vi "Estrai soglie.vi"(8 "error in (no error)":errorcluster, 10 "element":refnum<vi>) -> (0 "error out":errorcluster, 2 "Array soglie":T1(array[cluster]))   [LabVIEW 2019]
uses:
  <vilib>/Utility/file.llb/Read Delimited Spreadsheet (string).vi
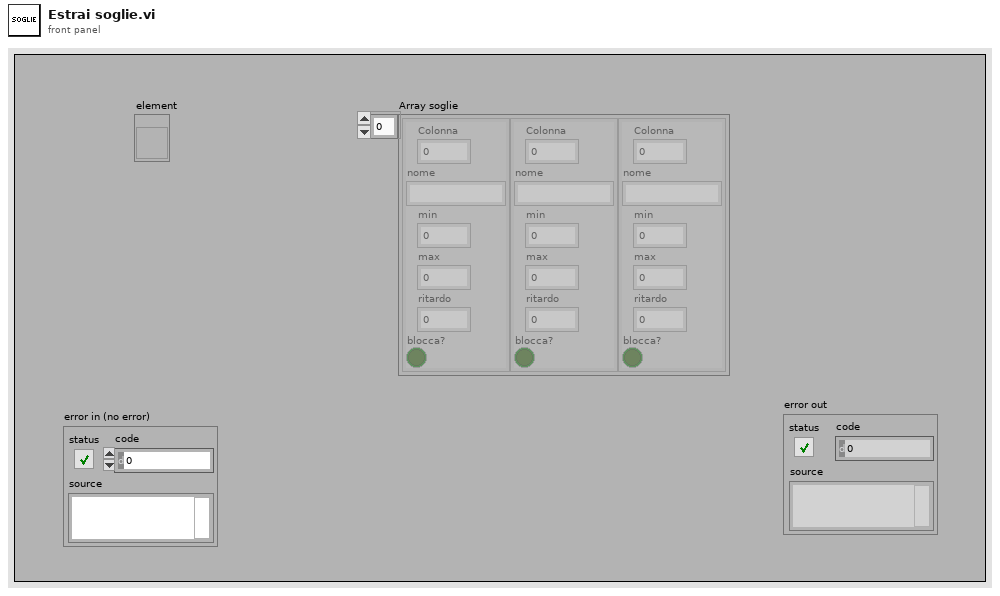
[diagram p1: front panel]
types:
  T1 = cluster{"Colonna":i16, "nome":string, "min":dbl, "max":dbl, "ritardo":dbl, "blocca?":bool}[]
  T2 = cluster{"Colonna":i16, "nome":string, "min":dbl, "max":dbl, "ritardo":dbl, "blocca?":bool}
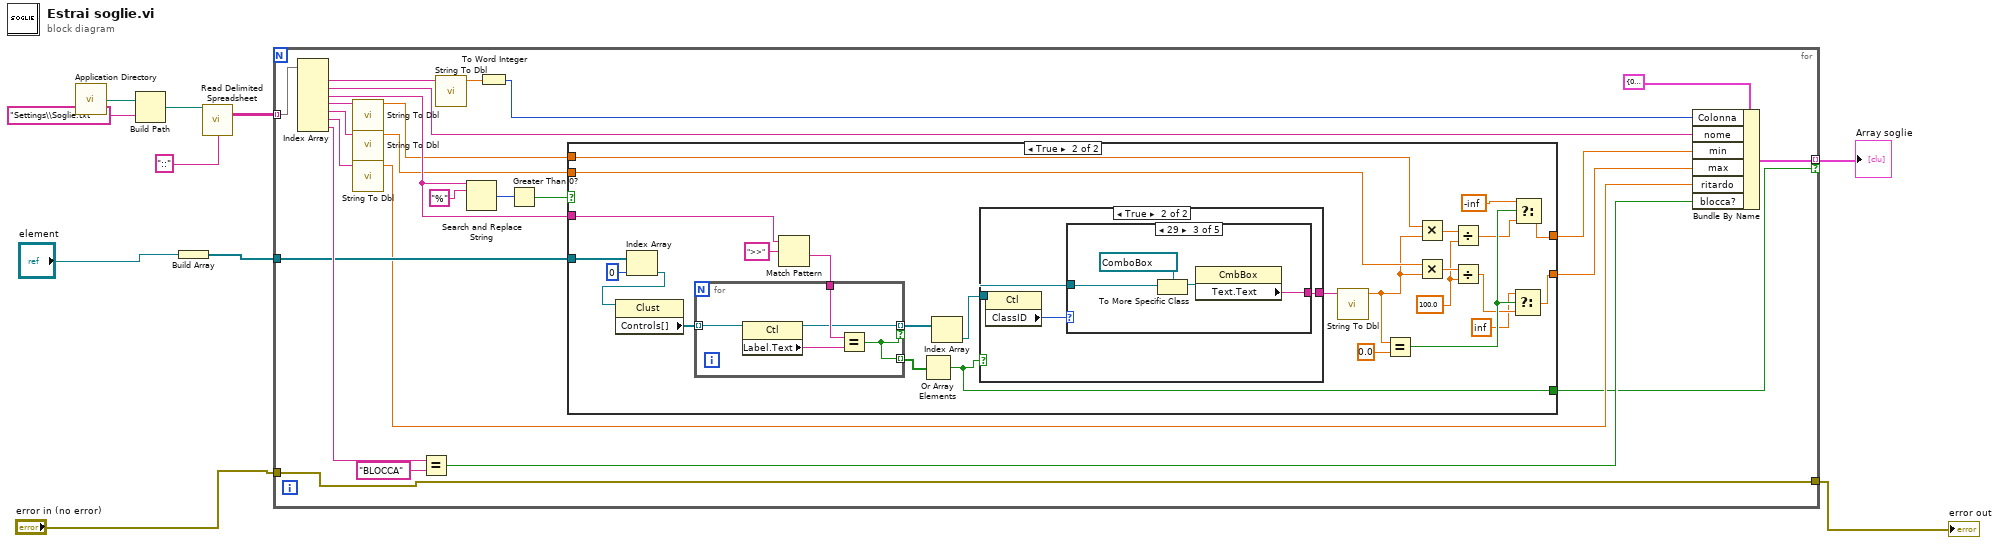
[diagram p0: block diagram]
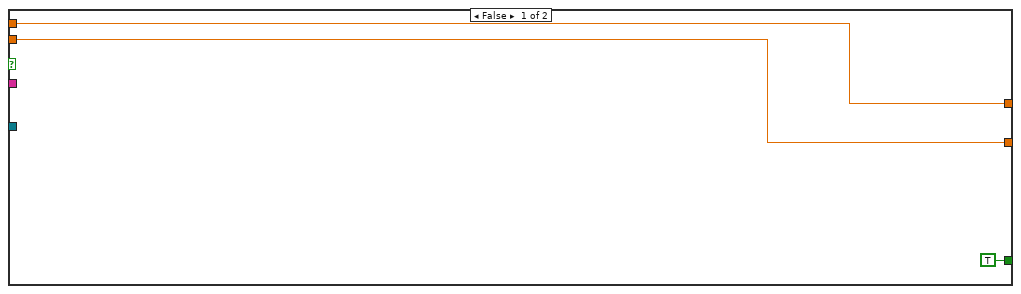
[diagram p2: hidden frame]
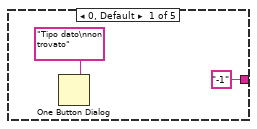
[diagram p4: hidden frame]
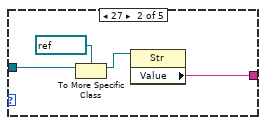
[diagram p5: hidden frame]
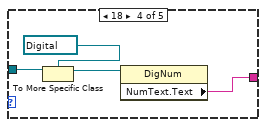
[diagram p6: hidden frame]
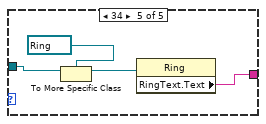
[diagram p7: hidden frame]
diagram:
  n1 = call <vilib>:"Application Directory.vi"() -> ("Application Directory"=w6:path)
  n2 = Build Path(base path=w6, name or relative path="Settings\\Soglie.txt") -> (appended path=w5:path)
  n3 = Build Array("element") -> (w10:refnum<vi>[])
  n4 = call-poly <vilib>:"Read Delimited Spreadsheet.vi"("file path (dialog if empty)"=w5, "delimiter (\\t)"="::" ("delimiter (\\t)")) -> ("all rows"=w9:string[][])  [unwired: 8 in, 5 out]
  n5 = for {
    tunnel: w9 -> [w35] mode=indexing
    tunnel: w10 -> [w24]
    tunnel: [w13] -> w4 mode=indexing if=w12
    tunnel: "error in (no error)" -> [w11]
    tunnel: [w11] -> w1
    n6 = Index Array(array=w35) -> (element #1=w34:string, element #2=w18:string, element #3=w23:string, element #4=w30:string, element #5=w29:string, element #6=w28:string, element #7=w27:string)  [unwired: 7 in]
    n7 = call "String To Dbl.vi"("String"=w30) -> ("Numeric"=w22:dbl)  [unwired: 10 in]
    n8 = call "String To Dbl.vi"("String"=w29) -> ("Numeric"=w21:dbl)  [unwired: 10 in]
    n9 = call "String To Dbl.vi"("String"=w28) -> ("Numeric"=w15:dbl)  [unwired: 10 in]
    n10 = Equal?(x=w27, y="BLOCCA") -> (x = y?=w14:bool)
    n11 = call "String To Dbl.vi"("String"=w34) -> ("Numeric"=w33:dbl)  [unwired: 10 in]
    n12 = Search and Replace String(input string=w23, search string="%") -> (number of replacements=w31:i32)  [unwired: 6 in, 3 out]
    n13 = To Word Integer(number=w33) -> (16bit integer=w19:i16)
    n14 = Greater Than 0?(x=w31) -> (x > 0?=w25:bool)
    n15 = case shown="True" w25 {
      tunnel: w24 -> [_ w64]
      tunnel: w23 -> [_ w42]
      tunnel: [w38 w45] -> w17
      tunnel: [w37 w46] -> w16
      tunnel: w22 -> [w38 w55]
      tunnel: w21 -> [w37 w54]
      tunnel: [TRUE w39] -> w12
      frame False {
      }
      frame True {
        w56 = 100.0 ("y")
        n16 = Index Array(array=w64, index=0) -> (element=w63:refnum<vi>)
        n17 = property class="Clust"(reference=w63) -> ("Controls[]"=w62:refnum<vi>[])  [unwired: 1 in, 2 out]
        n18 = Match Pattern(string=w42, regular expression=">>") -> (after substring=w41:string)  [unwired: 1 in, 3 out]
        n19 = for {
          tunnel: w62 -> [w90] mode=indexing
          tunnel: w41 -> [w88]
          tunnel: [w87] -> w61 mode=indexing if=w86
          tunnel: [w86] -> w40 mode=indexing
          n20 = property class="Ctl"(reference=w90) -> (reference out=w87:refnum<vi>, "Label.Text"=w89:string)  [unwired: 1 in, 1 out]
          n21 = Equal?(x=w88, y=w89) -> (x = y?=w86:bool)
        }
        n22 = Or Array Elements(Boolean array=w40) -> (logical OR=w39:bool)
        n23 = Index Array(array=w61) -> (element=w60:refnum<vi>)  [unwired: 1 in]
        n24 = case shown="True" w39 {
          tunnel: w60 -> [_ w67]
          tunnel: [_ w65] -> w59
          frame False {
          }
          frame True {
            n25 = property class="Ctl"(reference=w67) -> ("ClassID"=w66:u32)  [unwired: 1 in, 2 out]
            n26 = case shown="29" w66 {
              tunnel: w67 -> [_ w72 w75 w81 w84]
              tunnel: ["-1" ("RingText.Text") w70 w74 w78 w82] -> w65
              frame 0, Default {
                n27 = One Button Dialog(message="Tipo dato\nnon trovato") -> ()  [unwired: 1 in, 1 out]
              }
              frame 27 {
                n28 = To More Specific Class(target class=refnum<vi> refnum ("String"), reference=w72) -> (specific class reference=w71:refnum<vi>)  [unwired: 1 in, 1 out]
                n29 = property class="Str"(reference=w71) -> ("Value"=w70:string)  [unwired: 1 in, 2 out]
              }
              frame 29 {
                n30 = To More Specific Class(target class=refnum<vi> refnum ("String"), reference=w75) -> (specific class reference=w76:refnum<vi>)  [unwired: 1 in, 1 out]
                n31 = property class="CmbBox"(reference=w76) -> ("Text.Text"=w74:string)  [unwired: 1 in, 2 out]
              }
              frame 18 {
                n32 = To More Specific Class(target class=refnum<vi> refnum ("Numeric Control"), reference=w81) -> (specific class reference=w79:refnum<vi>)  [unwired: 1 in, 1 out]
                n33 = property class="DigNum"(reference=w79) -> ("NumText.Text"=w78:string)  [unwired: 1 in, 2 out]
              }
              frame 34 {
                n34 = To More Specific Class(target class=refnum<vi> refnum ("Menu Ring"), reference=w84) -> (specific class reference=w83:refnum<vi>)  [unwired: 1 in, 1 out]
                n35 = property class="Ring"(reference=w83) -> ("RingText.Text"=w82:string)  [unwired: 1 in, 2 out]
              }
            }
          }
        }
        n36 = call "String To Dbl.vi"("String"=w59) -> ("Numeric"=w53:dbl)  [unwired: 10 in]
        n37 = Equal?(x=w53, y=0.0) -> (x = y?=w51:bool)
        n38 = Multiply(x=w55, y=w53) -> (x*y=w58:dbl)
        n39 = Multiply(x=w54, y=w53) -> (x*y=w57:dbl)
        n40 = Divide(x=w58, y=w56) -> (x/y=w49:dbl)
        n41 = Divide(x=w57, y=w56) -> (x/y=w50:dbl)
        n42 = Select(t=inf ("y"), s=w51, f=w50) -> (s? t:f=w46:dbl)
        n43 = Select(t=-inf ("y"), s=w51, f=w49) -> (s? t:f=w45:dbl)
      }
    }
    n44 = Bundle By Name(cluster=T2 {"Colonna"=0, "nome"="", "min"=0.0, "max"=0.0, "ritardo"=0.0, "blocca?"=FALSE} ("output cluster"), "Colonna"=w19, "nome"=w18, "min"=w17, "max"=w16, "ritardo"=w15, "blocca?"=w14) -> (w13:T2)
  }
  "Array soglie" <- w4
  "error out" <- w1
